vi "SlowMotion.vi"() -> ()   [LabVIEW 2015]
panel:
  in  "Slow":bool
  in  "LastA":bool
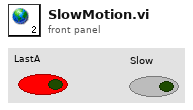
[diagram p1: front panel]
diagram:
